vi "distance_to_zeta.vi"(1 "D":dbl) -> (0 "wheel_zeta":dbl)   [LabVIEW 2017]
uses:
  Constant.vi
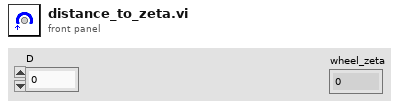
[diagram p1: front panel]
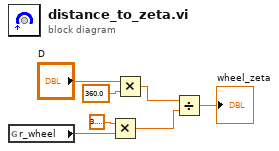
[diagram p0: block diagram]
diagram:
  n1 = global read "Constant.vi" "r_wheel"() -> (w4:dbl)
  n2 = Multiply(x=3.141592653589793, y=w4) -> (x*y=w2:dbl)
  n3 = Multiply(x="D", y=360.0) -> (x*y=w3:dbl)
  n4 = Divide(x=w3, y=w2) -> (x/y=→"wheel_zeta":dbl)
